vi "MPPT Silicon model NO ALGORITHM.vi"() -> ()   [LabVIEW 2017]
doc: "This example shows how to create, run a script and query the script output data."
panel:
  in  "Delay(ms)":u32=1000
  out "Current":dbl[](array[numeric])
  out "XY Graph":cluster{dbl[], dbl[]}[](graph)
  out "P(k-1)":dbl
  out "P(k)":dbl
  out "V(k-1)":dbl
  out "V(k)":dbl
  out "Voltage":dbl[](array[numeric])
  out "Power":dbl[](array[numeric])
  in  "stop":bool
  in  "dV":dbl=0.01 caption="limitI"
  in  "Initial Voltage (V)":dbl caption="limitI"
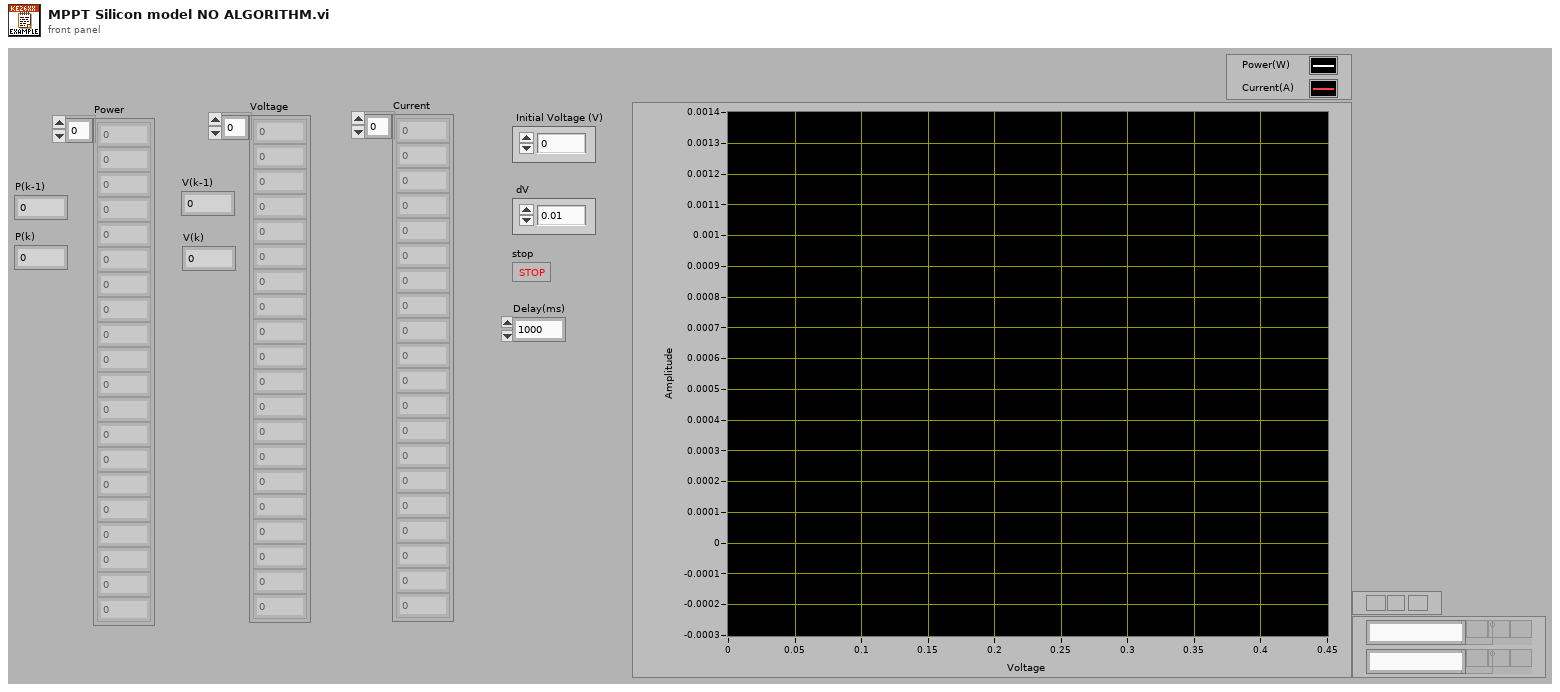
[diagram p1: front panel]
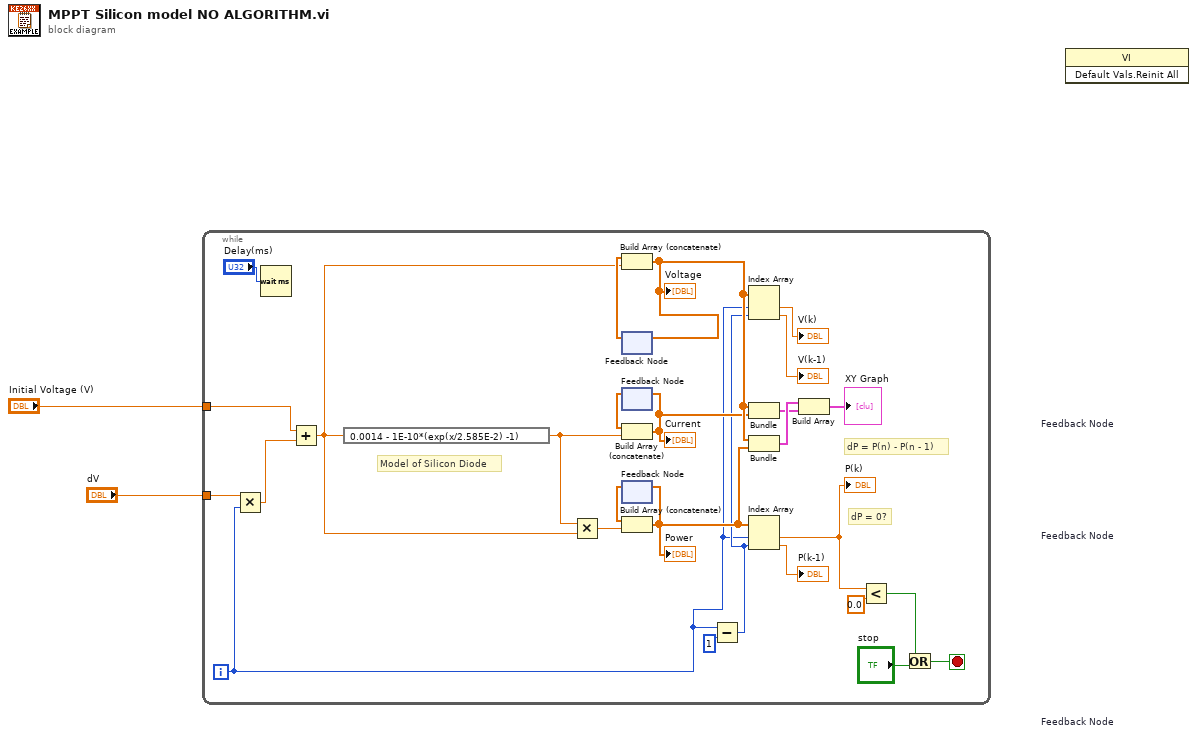
[diagram p0: block diagram]
diagram:
  n1 = while {
    tunnel: "dV" -> [w29]
    tunnel: "Initial Voltage (V)" -> [w27]
    i -> [w3]
    stop <- w6 stop-if-true
    # "dP = 0?"
    # "dP = P(n) - P(n - 1)"
    # "Model of Silicon Diode"
    n2 = Multiply(x=w29, y=w3) -> (x*y=w28:dbl)
    n3 = Wait (ms)(milliseconds to wait="Delay(ms)") -> ()  [unwired: 1 out]
    n4 = Add(x=w27, y=w28) -> (x+y=w12:dbl)
    n5 = expression code="0.0014 - 1E-10*(exp(x/2.585E-2) -1)"(w12) -> (w23:dbl)
    n6 = Multiply(x=w23, y=w12) -> (x*y=w25:dbl)
    n7 = feedback #1 "Feedback Node"() -> (w22:dbl[])  [unwired: 1 in]
    n8 = Build Array (concatenate)(w22, w12) -> (w20:dbl[])
    "Voltage" <- w20
    n9 = feedback-in #1(w20) -> ()
    n10 = feedback #2 "Feedback Node"() -> (w24:dbl[])  [unwired: 1 in]
    n11 = Build Array (concatenate)(w24, w23) -> (w13:dbl[])
    "Current" <- w13
    n12 = feedback-in #2(w13) -> ()
    n13 = feedback #3 "Feedback Node"() -> (w26:dbl[])  [unwired: 1 in]
    n14 = Build Array (concatenate)(w26, w25) -> (w21:dbl[])
    "Power" <- w21
    n15 = feedback-in #3(w21) -> ()
    n16 = Subtract(x=w3, y=1) -> (x-y=w10:i32)
    n17 = Index Array(array=w20, index #1=w3, index #2=w10) -> (element #1=→"V(k)":dbl, element #2=→"V(k-1)":dbl)
    n18 = Bundle(w20, w13) -> (w18:cluster{dbl[], dbl[]})  [unwired: 1 in]
    n19 = Bundle(w20, w21) -> (w19:cluster{dbl[], dbl[]})  [unwired: 1 in]
    n20 = Index Array(array=w21, index #1=w3, index #2=w10) -> (element #1=w7:dbl, element #2=→"P(k-1)":dbl)
    "P(k)" <- w7
    n21 = Build Array(w19, w18) -> (→"XY Graph":cluster{dbl[], dbl[]}[])
    n22 = Less?(x=w7, y=0.0) -> (x < y?=w4:bool)
    n23 = Or(x=w4, y="stop") -> (x .or. y?=w6:bool)
  }
  n24 = invoke class="VI" method="Default Vals.Reinit All"() -> ()  [unwired: 3 in, 3 out]
